vi "ACT_6_Task5_825005609.vi"() -> ()   [LabVIEW 2016]
panel:
  in  "Input 2":dbl
  in  "Input 1":dbl
  out "Output":dbl
  in  "Radio Buttons":T1(radio)
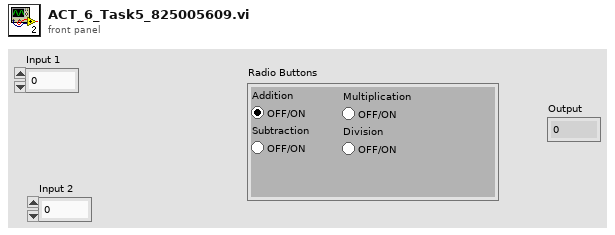
[diagram p1: front panel]
types:
  T1 = enum32{"Addition", "Subtraction", "Multiplication", "Division"}
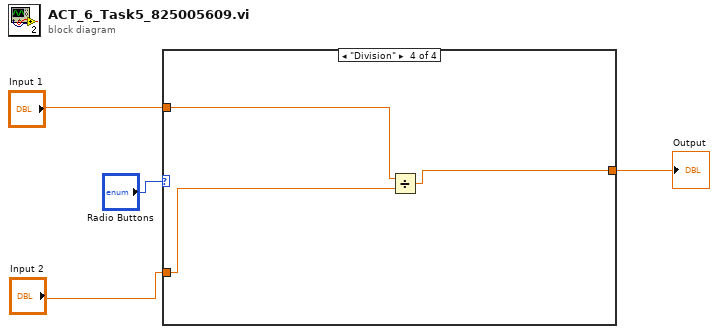
[diagram p0: block diagram]
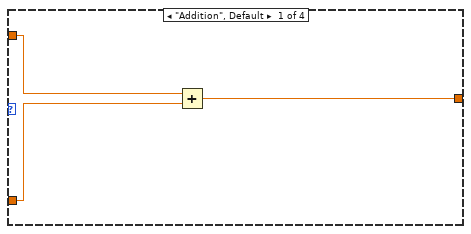
[diagram p2: hidden frame]
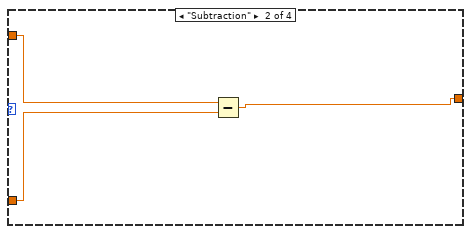
[diagram p3: hidden frame]
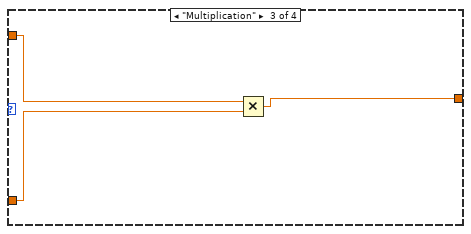
[diagram p4: hidden frame]
diagram:
  n1 = case shown="\"Division\"" "Radio Buttons" {
    tunnel: "Input 2" -> [w6 w9 w13 w15]
    tunnel: "Input 1" -> [w7 w10 w12 w16]
    tunnel: [w5 w8 w11 w14] -> w3
    frame "Addition", Default {
      n2 = Add(x=w7, y=w6) -> (x+y=w5:dbl)
    }
    frame "Subtraction" {
      n3 = Subtract(x=w10, y=w9) -> (x-y=w8:dbl)
    }
    frame "Multiplication" {
      n4 = Multiply(x=w12, y=w13) -> (x*y=w11:dbl)
    }
    frame "Division" {
      n5 = Divide(x=w16, y=w15) -> (x/y=w14:dbl)
    }
  }
  "Output" <- w3
